vi "SetStrArrToRingCtrl.vi"(10 "str arr":string[](array[string]), 11 "ref in":refnum<vi>) -> (3 "ref out":refnum<vi>)   [LabVIEW 2018, in "Library-Ctrl.lvlib"]
uses:
  Library-Ctrl.lvlib
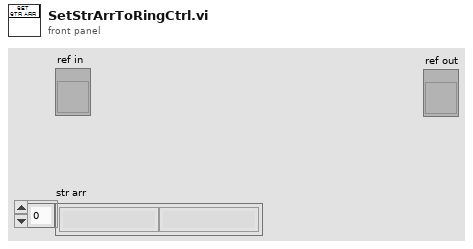
[diagram p1: front panel]
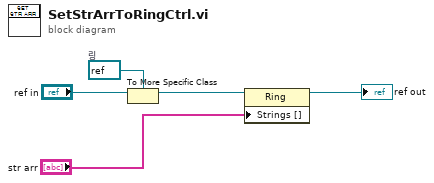
[diagram p0: block diagram]
diagram:
  w1 = refnum<vi> refnum  # 링
  n1 = To More Specific Class(target class=w1, reference="ref in") -> (specific class reference=w2:refnum<vi>)  [unwired: 1 in, 1 out]
  n2 = property class="Ring"(reference=w2, "Strings []"="str arr") -> (reference out=→"ref out":refnum<vi>)  [unwired: 1 in, 1 out]
